vi "checksum.vi"(8 "error in (no error)":errorcluster, 10 "input":string, 11 "EMTestCWS500N in":refnum<class "EMTestCWS500N.lvclass">) -> (0 "error out":errorcluster, 2 "output":string, 3 "EMTestCWS500N out":refnum<class "EMTestCWS500N.lvclass">)   [LabVIEW 2013, in "EMTestCWS500N.lvclass"]
uses:
  EMTestCWS500N.lvclass
  dll/libchecksum.dll
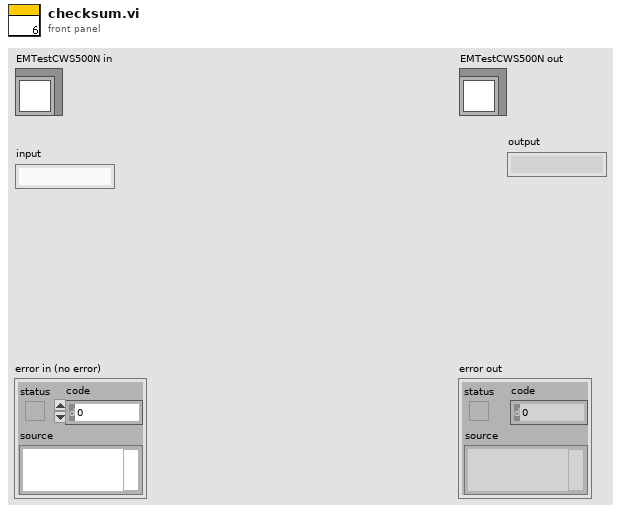
[diagram p1: front panel]
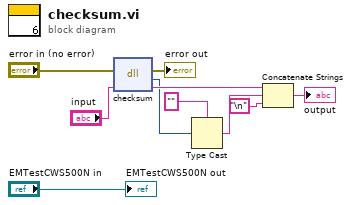
[diagram p0: block diagram]
diagram:
  n1 = dll-call lib="H:/sze/Bachelor Thesis/resourcen/Hauptprojekt/EMV/res/dll/libchecksum.dll" fn="checksum"(error in="error in (no error)", "befehl"="input") -> (error out=→"error out":errorcluster, "checksum"=w8:u8, "befehl"=w9:string)  [unwired: 2 in, 1 out]
  n2 = Type Cast(type="", x=w8) -> (*(type *) &x=w10:string)
  n3 = Concatenate Strings(w9, w10, "\n") -> (→"output":string)
  "EMTestCWS500N out" <- "EMTestCWS500N in"
